vi "S8300E_NETLink_Speed_WIH.vi"() -> ()   [LabVIEW 2011]
panel:
  out "PRELOG2":string
  out "PRELOG1":string
  out "LOG Message":string
  out "VISA resource name out":refnum<visa-resource-name>
  out "cmd list":T1(array[cluster])
  out "PORT3 SPEED":string
  out "PORT2 SPEED":string
  out "PORT1 SPEED":string
  out "進行狀況":string
  out "BEGIN TIME":u32
  # "S8300E Check 3 NET PORTs Link ,Speed"
  # "2015-6-1"
  # "Error Code:PORT1LS\nError Code:PORT2LS\nError Code:PORT3LS"
  # "Step1:PORT1 LINK\nStep2:PORT1 Speed\nStep3:PORT2 LINK\nStep4:PORT2 Speed\nStep5:PORT3 LINK\nStep6:PORT3 Speed"
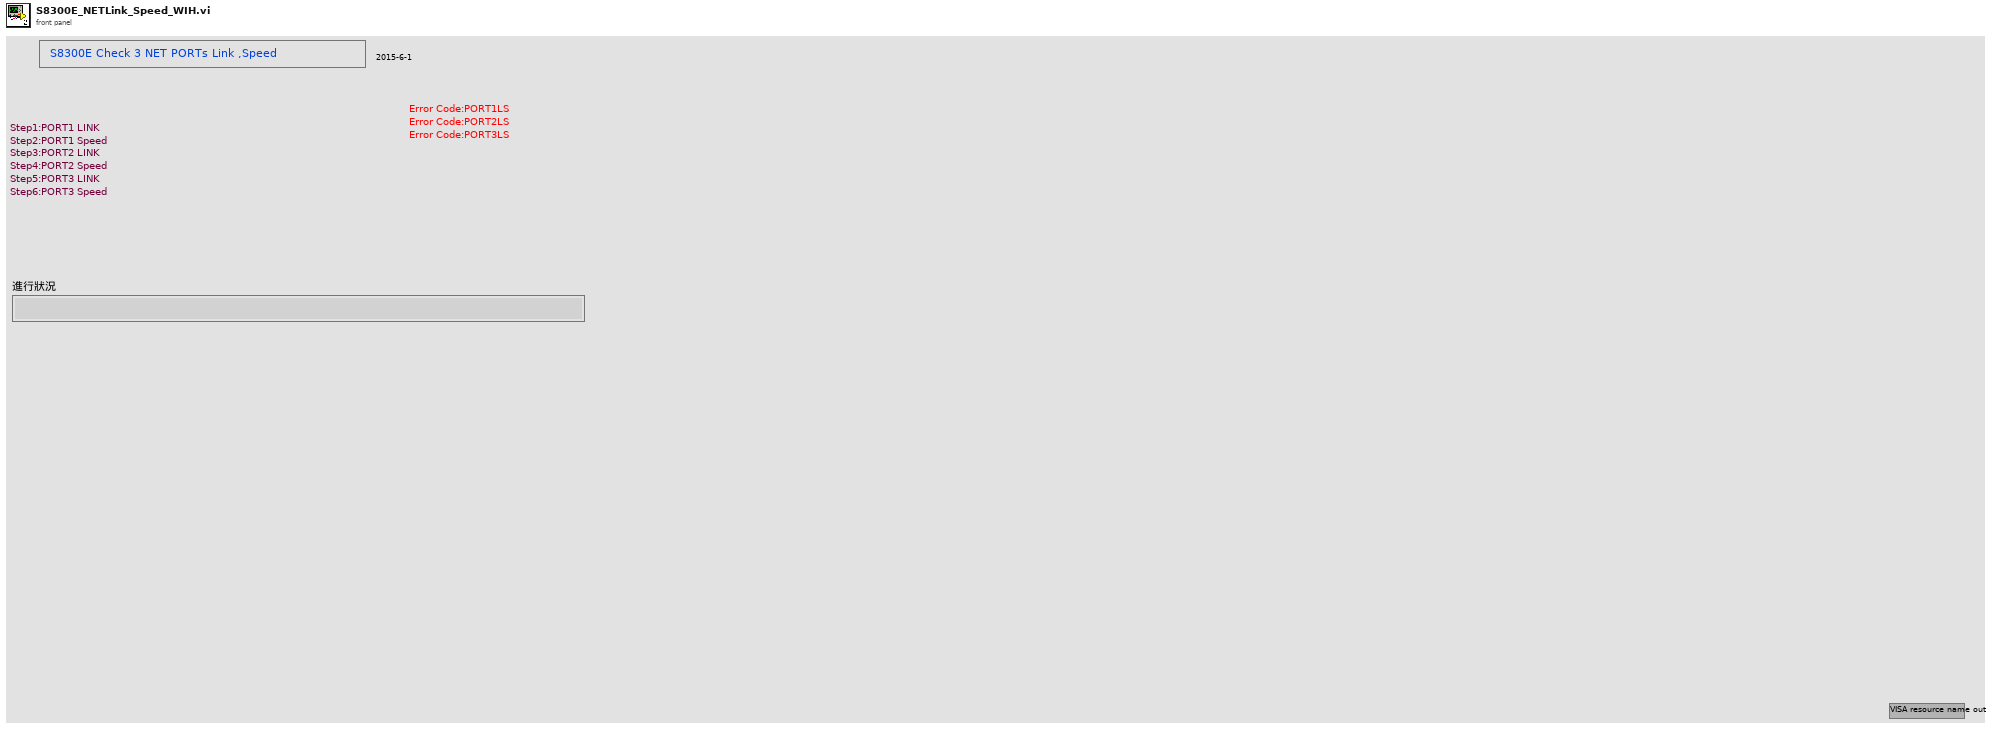
[diagram p1: front panel]
types:
  T1 = cluster{"cmd":string, "Pass String":string, "Msg status":string, "Error Code":string}[]
  T2 = cluster{"cmd":string, "Pass String":string, "Msg status":string, "Error Code":string}
  T3 = cluster{"cmd":string, string, "Msg status":string, "Error Code":string}
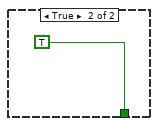
[diagram p5: hidden frame]
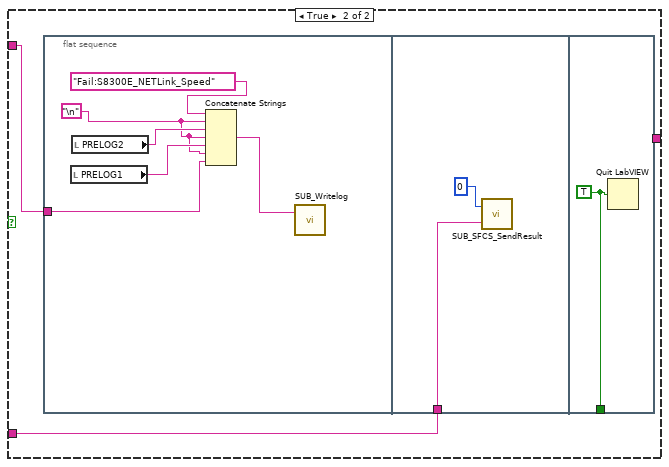
[diagram p6: hidden frame]
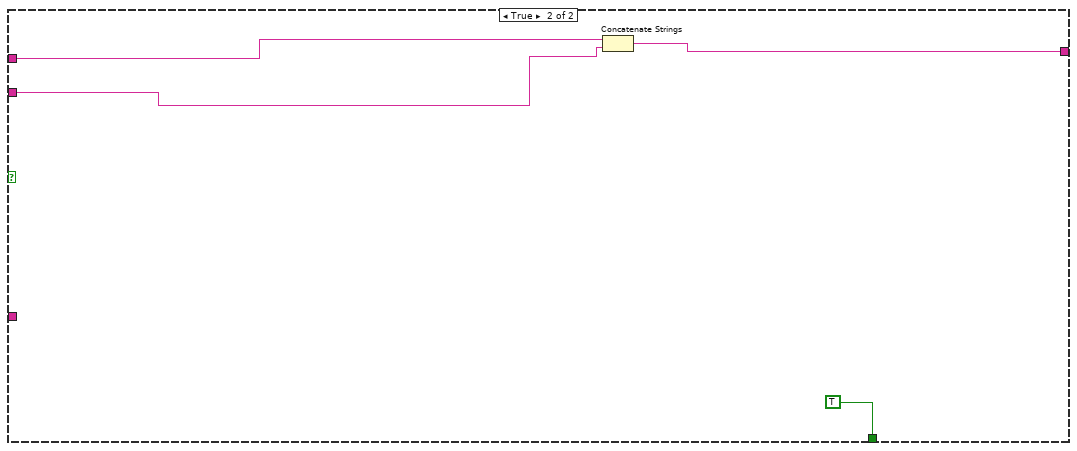
[diagram p7: hidden frame]
diagram:
  n1 = flat-sequence {
    frame #0 {
      n2 = Tick Count (ms)() -> (millisecond timer value=→"BEGIN TIME":u32)
    }
    frame #1 {
      w2 = ""
      n3 = local write "PORT2 SPEED"(w2) -> ()
      n4 = local write "PORT3 SPEED"(w2) -> ()
      n5 = local write "PORT1 SPEED"(w2) -> ()
      n6 = property on="進行狀況" class="Str"("Blinking"=TRUE) -> ()  [unwired: 2 in, 2 out]
      "進行狀況" <- "進入測試準備中...." ("進行狀況")
    }
    frame #2 {
      w5 = "1000MB"
      n7 = local write "PORT1 SPEED"(w5) -> ()
      n8 = local write "PORT2 SPEED"(w5) -> ()
      n9 = local write "PORT3 SPEED"(w5) -> ()
    }
    frame #3 {
      n10 = call "SUB_ReadScript_File.vi"("Script FileName"="S8300E_sfcs_misc.txt" ("Search Filename in Folder")) -> ("text"=w14:string)  [unwired: 1 in, 2 out]
      n11 = call "SUB_FindSpecificString.vi"("Find this String"="UUT_PORT2_LINK_SPEED=", "String data"=w14) -> ("before \"; \" string"=→"PORT2 SPEED":string, "Found"=w12:bool)  [unwired: 2 in]
      n12 = call "SUB_FindSpecificString.vi"("Find this String"="UUT_PORT3_LINK_SPEED=", "String data"=w14) -> ("before \"; \" string"=→"PORT3 SPEED":string, "Found"=w10:bool)  [unwired: 2 in]
      n13 = call "SUB_FindSpecificString.vi"("Find this String"="UUT_PORT1_LINK_SPEED=", "String data"=w14) -> ("before \"; \" string"=→"PORT1 SPEED":string, "Found"=w13:bool)  [unwired: 2 in]
      n14 = And(x=w13, y=w12) -> (x .and. y?=w11:bool)
      n15 = And(x=w11, y=w10) -> (x .and. y?=w9:bool)
      n16 = case shown="False" w9 {
        frame False {
          n17 = flat-sequence {
            frame #0 {
              n18 = call "Display Message to User"() -> ()  [unwired: 10 in, 2 out]
            }
            frame #1 {
              n19 = call "SUB_Writelog.vi"("Pass/Fail"="Fail:S8300E_NETLink_Speed") -> ()  [unwired: 2 in]
            }
            frame #2 {
              n20 = Quit LabVIEW(quit? (T)=TRUE) -> ()
            }
          }
        }
        frame True {
        }
      }
    }
    frame #4 {
      w31 = "PORT3LS"  # Error Code
      w32 = "Checking PORT3 Speed  function"  # Msg status
      w30 = "PASSED="  # Pass String
      w33 = "./eth.sh -p 3"  # cmd
      w34 = "PORT3LS"  # Error Code
      w35 = "Checking PORT3  Link function"  # Msg status
      w36 = "PASSED=Linked"  # Pass String
      w37 = "./eth.sh -s 3"  # cmd
      w41 = "PORT2LS"  # Error Code
      w42 = "Checking PORT2 Speed  function"  # Msg status
      w40 = "PASSED="  # Pass String
      w43 = "./eth.sh -p 2"  # cmd
      w44 = "PORT2LS"  # Error Code
      w45 = "Checking PORT2  Link function"  # Msg status
      w46 = "PASSED=Linked"  # Pass String
      w47 = "./eth.sh -s 2"  # cmd
      w51 = "PORT1LS"  # Error Code
      w52 = "Checking PORT1 Speed  function"  # Msg status
      w50 = "PASSED="  # Pass String
      w53 = "./eth.sh -p 1"  # cmd
      w54 = "PORT1LS"  # Error Code
      w55 = "Checking PORT1 Link function"  # Msg status
      w56 = "PASSED=Linked"  # Pass String
      w57 = "./eth.sh -s 1"  # cmd
      n21 = local read "PORT3 SPEED"() -> (w28:string)
      n22 = local read "PORT2 SPEED"() -> (w38:string)
      n23 = local read "PORT1 SPEED"() -> (w49:string)
      n24 = Concatenate Strings(w40, w38) -> (w39:string)
      n25 = Concatenate Strings(w50, w49) -> (w48:string)
      n26 = Concatenate Strings(w30, w28) -> (w29:string)
      n27 = Bundle("cmd"=w47, "Pass String"=w46, "Msg status"=w45, "Error Code"=w44) -> (w25:T2)  [unwired: 1 in]
      n28 = Bundle("cmd"=w57, "Pass String"=w56, "Msg status"=w55, "Error Code"=w54) -> (w27:T2)  [unwired: 1 in]
      n29 = Bundle("cmd"=w37, "Pass String"=w36, "Msg status"=w35, "Error Code"=w34) -> (w23:T2)  [unwired: 1 in]
      n30 = Bundle("cmd"=w43, w39, "Msg status"=w42, "Error Code"=w41) -> (w24:T3)  [unwired: 1 in]
      n31 = Bundle("cmd"=w53, w48, "Msg status"=w52, "Error Code"=w51) -> (w26:T3)  [unwired: 1 in]
      n32 = Bundle("cmd"=w33, w29, "Msg status"=w32, "Error Code"=w31) -> (w22:T3)  [unwired: 1 in]
      n33 = Build Array(w27, w26, w25, w24, w23, w22) -> (→"cmd list":T1)
    }
    frame #5 {
      n34 = call "SUB_COM1_CLOSE.vi"("VISA resource name"=refnum<visa-resource-name> "COM9") -> ()  [unwired: 3 in]
    }
    frame #6 {
      n35 = case shown="True" TRUE {
        frame False {
        }
        frame True {
          n36 = call "SUB_COM9_INIT.vi"("baud rate"=u32 115200) -> ("VISA resource name out"=w63:refnum<visa-resource-name>)  [unwired: 1 in, 1 out]
          "VISA resource name out" <- w63
          n37 = call "SUB_COM1Wrt.vi"("VISA resource name"=w63, "write buffer"="\r") -> ("duplicate VISA resource name"=w60:refnum<visa-resource-name>)  [unwired: 1 in, 1 out]
          n38 = call "SUB_ContinueCom1Read.vi"("Numeric"=1200, "duplicate VISA resource name 2"=w60) -> ()  [unwired: 1 in, 3 out]
        }
      }
    }
    frame #7 {
      n39 = while {
        stop <- w74 stop-if-true
        w70 = "S8300E" ("Find this String")
        n40 = local read "VISA resource name out"() -> (w66:refnum<visa-resource-name>)
        n41 = Tick Count (ms)() -> (millisecond timer value=w72:u32)
        n42 = call "SUB_ContinueCom1Read.vi"("Numeric"=1200, "duplicate VISA resource name 2"=w66) -> ("duplicate VISA resource name"=w65:refnum<visa-resource-name>)  [unwired: 1 in, 2 out]
        n43 = call "SUB_COM1Wrt.vi"("VISA resource name"=w65, "write buffer"="\r") -> ("duplicate VISA resource name"=w73:refnum<visa-resource-name>)  [unwired: 1 in, 1 out]
        n44 = call "SUB_READ_COM1_FindString_timeout.vi"("Find this String"=w70, "Timeout Seccond"=3.0, "Begin time"=w72, "duplicate VISA resource name 2"=w73) -> ("Output String"=w69:string)  [unwired: 1 in, 2 out]
        n45 = call "SUB_FindSpecificString.vi"("Find this String"=w70, "String data"=w69) -> ("Found"=w68:bool)  [unwired: 2 in, 1 out]
        n46 = case shown="False" w68 {
          tunnel: [w77 TRUE] -> w74
          tunnel: w69 -> [w76 _]
          frame False {
            n47 = call "SUB_YESNO.vi"("Debug View"=w76, "Status"="UART無正確反應!需有S8300E字串") -> ("yes/no"=w80:enum32{"No Selection", "Yes", "No", "None"})  [unwired: 1 in]
            n48 = Equal?(x=w80, y=enum32{"No Selection", "Yes", "No", "None"}."No") -> (x = y?=w78:bool)
            n49 = case shown="True" w78 {
              tunnel: [_ w82] -> w77
              frame False {
              }
              frame True {
                n50 = flat-sequence {
                  tunnel: [w86] -> w82
                  frame #0 {
                    n51 = call "SUB_Writelog.vi"("Pass/Fail"="Fail:S8300E_NETLink_Speed") -> ()  [unwired: 2 in]
                  }
                  frame #1 {
                    n52 = call "SUB_SFCS_SendResult.vi"("ErrorCode"="UART", "PASS_Fail (1/0)"=i8 0) -> ()  [unwired: 1 out]
                  }
                  frame #2 {
                    w86 = TRUE ("quit? (T)")
                    n53 = Quit LabVIEW(quit? (T)=w86) -> ()
                  }
                }
              }
            }
          }
          frame True {
          }
        }
      }
    }
    frame #8 {
      n54 = local read "cmd list"() -> (w91:T1)
      n55 = Array Size(array=w91) -> (size(s)=w90:i32)
      n56 = for {
        N: w90 -> [_]
        shift-right: [w93] -> w88
        shift-left: "" -> [w92]
        i -> [w96]
        n57 = while {
          tunnel: w96 -> [w116]
          shift-right: [w100] -> w94
          shift-left: "" -> [w99]
          stop <- w106 stop-if-true
          n58 = local read "cmd list"() -> (w117:T1)
          n59 = local read "VISA resource name out"() -> (w102:refnum<visa-resource-name>)
          n60 = Index Array(array=w117, index=w116) -> (element=w115:T2)
          n61 = call "SUB_ContinueCom1Read.vi"("Numeric"=1200, "duplicate VISA resource name 2"=w102) -> ("duplicate VISA resource name"=w101:refnum<visa-resource-name>)  [unwired: 1 in, 2 out]
          n62 = Unbundle By Name(w115) -> ("cmd"=w113:string, "Pass String"=w104:string, "Msg status"=w114:string, "Error Code"=w107:string)
          n63 = Concatenate Strings(w113, "\r") -> (w97:string)
          n64 = local write "進行狀況"(w114) -> ()
          n65 = Tick Count (ms)() -> (millisecond timer value=w111:u32)
          n66 = call "SUB_COM1Wrt.vi"("VISA resource name"=w101, "write buffer"=w97) -> ("duplicate VISA resource name"=w105:refnum<visa-resource-name>)  [unwired: 1 in, 1 out]
          n67 = call "SUB_READ_COM1_FindString_timeout.vi"("Find this String"=w104, "Timeout Seccond"=2.0, "Begin time"=w111, "duplicate VISA resource name 2"=w105) -> ("Output String"=w108:string, "Found String"=w109:bool)  [unwired: 1 in, 1 out]
          n68 = case shown="False" w109 {
            tunnel: w108 -> [w121 w145]
            tunnel: w107 -> [w126 _]
            tunnel: [_ TRUE] -> w106
            tunnel: [w119 w144] -> w98
            tunnel: w104 -> [w124 _]
            tunnel: w97 -> [_ w143]
            frame False {
              w120 = "\n"
              n69 = local read "進行狀況"() -> (w125:string)
              n70 = Concatenate Strings("測試失敗!系統需回 " ("string"), w124, "\r", w125) -> (w122:string)
              n71 = call "SUB_YESNO.vi"("Debug View"=w121, "Status"=w122) -> ("yes/no"=w129:enum32{"No Selection", "Yes", "No", "None"})  [unwired: 1 in]
              n72 = Equal?(x=w129, y=enum32{"No Selection", "Yes", "No", "None"}."No") -> (x = y?=w127:bool)
              n73 = Concatenate Strings(w122, w120, w121, w120) -> (w118:string)
              n74 = case shown="False" w127 {
                tunnel: w126 -> [_ w133]
                tunnel: [w131 _] -> w119
                tunnel: w118 -> [w131 w132]
                frame False {
                }
                frame True {
                  n75 = flat-sequence {
                    tunnel: w132 -> [w134]
                    tunnel: w133 -> [w140]
                    tunnel: [w142] -> _
                    frame #0 {
                      w136 = "\n"
                      n76 = local read "PRELOG1"() -> (w137:string)
                      n77 = local read "PRELOG2"() -> (w138:string)
                      n78 = Concatenate Strings("Fail:S8300E_NETLink_Speed" ("Pass/Fail"), w136, w138, w136, w137, w136, w134) -> (w135:string)
                      n79 = call "SUB_Writelog.vi"("Pass/Fail"=w135) -> ()  [unwired: 2 in]
                    }
                    frame #1 {
                      n80 = call "SUB_SFCS_SendResult.vi"("ErrorCode"=w140, "PASS_Fail (1/0)"=i8 0) -> ()  [unwired: 1 out]
                    }
                    frame #2 {
                      w142 = TRUE ("quit? (T)")
                      n81 = Quit LabVIEW(quit? (T)=w142) -> ()
                    }
                  }
                }
              }
            }
            frame True {
              n82 = Concatenate Strings(w143, w145) -> (w144:string)
            }
          }
          n83 = Concatenate Strings(w99, w98) -> (w100:string)
          "PRELOG1" <- w100
        }
        n84 = Concatenate Strings(w92, w94) -> (w93:string)
        "PRELOG2" <- w93
      }
      "LOG Message" <- w88
    }
    frame #9 {
      n85 = call "SUB_COM1_CLOSE.vi"("VISA resource name"=refnum<visa-resource-name> "COM9") -> ()  [unwired: 3 in]
    }
    frame #10 {
      w150 = "***Not Good ***" ("replace string (\"\")")
      w155 = "\r"
      n86 = Tick Count (ms)() -> (millisecond timer value=w157:u32)
      n87 = local read "BEGIN TIME"() -> (w158:u32)
      n88 = local read "LOG Message"() -> (w159:string)
      n89 = call "SUB_CAL_TESTTIME.vi"("Test Item name"="S8300E_NETLink_Speed", "Stop tick time"=w157, "Start tick time"=w158) -> ("Test Time output"=w154:string)  [unwired: 2 in]
      n90 = Concatenate Strings("Pass:S8300E_NETLink_Speed" ("string"), w155, w159, w155, w154) -> (w149:string)
      n91 = call "SUB_SEARCH_REPLACE_STR.vi"("replace string (\"\")"=w150, "search string"="FAILED", "input string"=w149) -> ("result string"=w152:string)  [unwired: 2 in]
      n92 = call "SUB_SEARCH_REPLACE_STR.vi"("replace string (\"\")"=w150, "search string"="FAIL", "input string"=w152) -> ("result string"=w148:string)  [unwired: 2 in]
      n93 = call "SUB_Writelog.vi"("Pass/Fail"=w148) -> ()  [unwired: 2 in]
    }
    frame #11 {
      n94 = Request Deallocation(TRUE ("flag")) -> ()
    }
    frame #12 {
      n95 = Quit LabVIEW(quit? (T)=TRUE) -> ()
    }
  }
